vi "Get Build Types.vi"(11 "CD Build Tools in":refnum<class "Project Build Tools.lvclass">) -> (2 "Build Types":T1[](array[typedef]), 3 "CD Build Tools out":refnum<class "Project Build Tools.lvclass">)   [LabVIEW 2019, in "Project Build Tools.lvclass"]
uses:
  Project Build Tools.lvclass
  TypeDefs/Configure Build Types.ctl
  Project Build Tools.lvclass/Project Build Tools.ctl
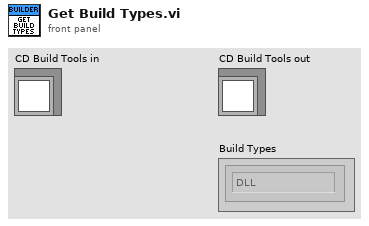
[diagram p1: front panel]
types:
  T1 = typedef "Project Build Tools.lvclass/Configure Build Types.ctl" = enum16{"DLL", "Packed Library", "Installer", "Source Distribution", "EXE"}
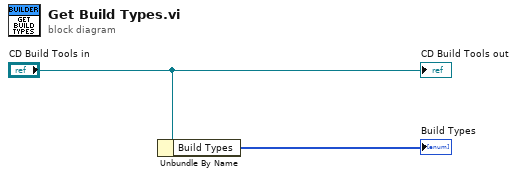
[diagram p0: block diagram]
diagram:
  n1 = Unbundle By Name("CD Build Tools in") -> ("Build Types"=→"Build Types":T1[])
  "CD Build Tools out" <- "CD Build Tools in"
